vi "Digital Signals Control.vi"(8 "error in":errorcluster, 9 "Device Inputs":dbl[](array[numeric]), 10 "DCM Ref":refnum<class "DCM - RT.lvclass">, 11 "Digital Signals":T1={"FIFO Indexes"={"Write"={"User OS"=0, "User OS Time [s]"=0}}, "Settings"={"Diff IO Filters [s]"=[0.0, 0.0, 0.0, 0.0, 0.0, 0.0, 0.0, 0.0], "Aux In Filters [s]"=[0.0, 0.0, 0.0, 0.0, 0.0, 0.0, 0.0, 0.0], "Serial In 1"=enum."Unused", "Serial In 2"=enum."Unused"}} {"Settings"."Aux In Filters [s]" min=0; "Settings"."Diff IO Filters [s]" min=0}) -> (0 "error out":errorcluster)   [LabVIEW 2016, in "DCM Engine.lvlib"]
uses:
  DCM Engine.lvlib
  Built/DCM Classes Packed/Pharlap/C/DCM-Classes.lvlibp/DCM/Rev0/RT/DCM - RT.lvclass
  Shared/Types/Digital Signals.ctl
  Built/DCM Classes Packed/Pharlap/C/DCM-Classes.lvlibp/1abvi3w/vi.lib/Powertrain Controls/Device Drivers/DCM/Rev0/FPGA/Digital Channel.ctl
  Built/DCM Classes Packed/Pharlap/C/DCM-Classes.lvlibp/DCM/Tools/RT/DCM - RT - Tools.lvlib
  DCM Shared.lvlib
  Built/DCM Classes Packed/Pharlap/C/DCM-Classes.lvlibp/1abvi3w/vi.lib/Powertrain Controls/Device Drivers/DCM/Rev0/FPGA/DCM - FPGA.lvlib
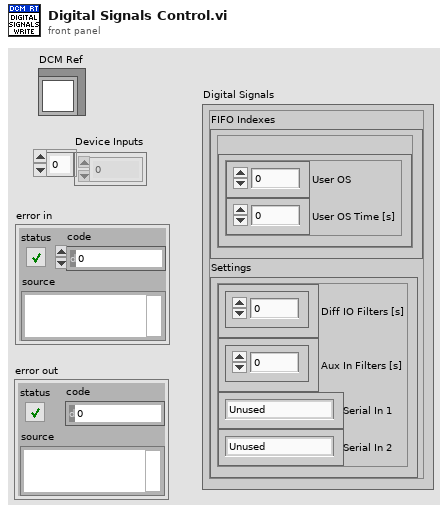
[diagram p1: front panel]
types:
  T1 = typedef "DCM Shared.lvlib/Digital Signals.ctl" = cluster{"FIFO Indexes":cluster{"Write":cluster{"User OS":i32, "User OS Time [s]":i32}}, "Settings":cluster{"Diff IO Filters [s]":sgl[], "Aux In Filters [s]":sgl[], "Serial In 1":T2, "Serial In 2":T2}}
  T2 = typedef "DCM-Classes.lvlibp/DCM - FPGA.lvlib/Digital Channel.ctl" = enum8{"Unused", "User OS", "Diff IO 1", "Diff IO 2", "Diff IO 3", "Diff IO 4", "Diff IO 5", "Diff IO 6", "Diff IO 7", "Diff IO 8", "Aux 1", "Aux 2", "Aux 3", "Aux 4", "Aux 5", "Aux 6", "Aux 7", "Aux 8", "Aux 9", "Aux 10", "Aux 11", "Aux 12", "Aux 13", "Aux 14", "Aux 15", "Aux 16"}
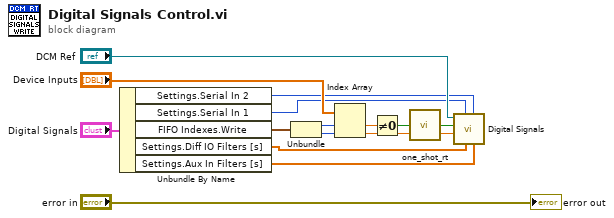
[diagram p0: block diagram]
diagram:
  n1 = Unbundle By Name("Digital Signals") -> ("Settings.Serial In 2"=w2:T2, "Settings.Serial In 1"=w1:T2, "FIFO Indexes.Write"=w11:cluster{"User OS":i32, "User OS Time [s]":i32}, "Settings.Diff IO Filters [s]"=w4:sgl[], "Settings.Aux In Filters [s]"=w3:sgl[])
  n2 = Unbundle(w11) -> ("User OS"=w10:i32, "User OS Time [s]"=w9:i32)
  n3 = Index Array(array="Device Inputs", index #1=w10, index #2=w9) -> (element #1=w8:dbl, element #2=w7:dbl)
  n4 = Not Equal To 0?(x=w8) -> (x != 0?=w6:bool)
  n5 = call <vilib>:"one_shot_rt.vi"("I"=w6) -> ("O"=w5:bool)
  n6 = call "Digital Signals.vi"("Aux In Filters [s]"=w3, "Serial In 2"=w2, "Diff IO Filters [s]"=w4, "Serial In 1"=w1, "User OS Time [s]"=w7, "User OS"=w5, "DCM Reference"="DCM Ref") -> ()  [unwired: 5 in]
  "error out" <- "error in"
